vi "Excel_Page_Setup.vi"(0 "Excel._Worksheet":refnum<k7>, 5 "Excel._Application":refnum<k7>, 7 "margins (1.00)":T1 {"bottom" format="%0.2f"; "right" format="%0.2f"; "left" format="%0.2f"; "top" format="%0.2f"}, 9 "measurement system (Default)":u16, 11 "error in (no error)":errorcluster) -> (15 "error out":errorcluster)   [LabVIEW 2017, in "NI_ReportGenerationToolkit.lvlib"]
uses:
  <vilib>/addons/_office/NI_ReportGenerationToolkit.lvlib
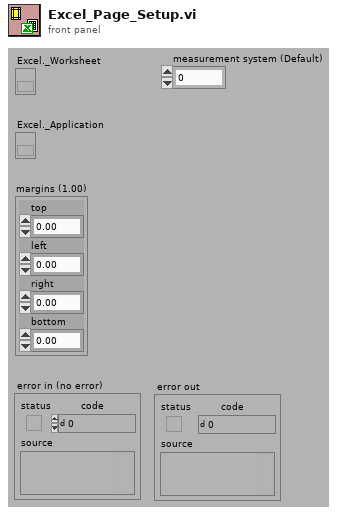
[diagram p1: front panel]
types:
  T1 = cluster{"top":dbl, "left":dbl, "right":dbl, "bottom":dbl}
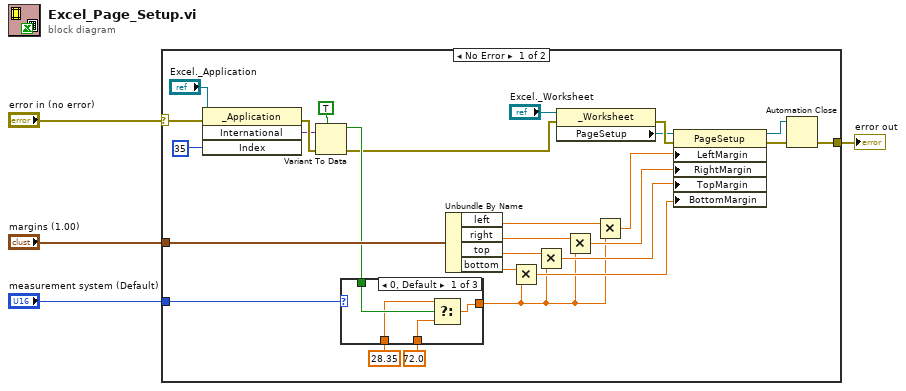
[diagram p0: block diagram]
diagram:
  n1 = case shown="No Error" "error in (no error)" {
    selector: "error in (no error)" -> [w5 w38]
    tunnel: "margins (1.00)" -> [w31 _]
    tunnel: "measurement system (Default)" -> [w11 _]
    tunnel: [w10 w38] -> w2
    frame No Error {
      n2 = invoke class="_Application" method="International"(reference="Excel._Application", error in=w5, "Index"=35) -> (error out=w21:errorcluster, "International"=w20:variant)  [unwired: 1 in, 2 out]
      n3 = Variant To Data(error in=w21, type=TRUE, Variant=w20) -> (data=w24:bool, error out=w22:errorcluster)
      n4 = case shown="0, Default" w11 {
        tunnel: [w35 w36 w37] -> w12
        tunnel: 72.0 -> [w32 w36 _]
        tunnel: w24 -> [w34 _ _]
        tunnel: 28.35 -> [w33 _ w37]
        frame 0, Default {
          n5 = Select(t=w33, s=w34, f=w32) -> (s? t:f=w35:dbl)
        }
        frame 1 {
        }
        frame 2 {
        }
      }
      n6 = Unbundle By Name(w31) -> ("left"=w30:dbl, "right"=w29:dbl, "top"=w28:dbl, "bottom"=w27:dbl)
      n7 = Multiply(x=w27, y=w12) -> (x*y=w16:dbl)
      n8 = Multiply(x=w28, y=w12) -> (x*y=w15:dbl)
      n9 = property class="_Worksheet"(reference="Excel._Worksheet", error in=w22) -> (error out=w9:errorcluster, "PageSetup"=w6:refnum<k7>)  [unwired: 1 out]
      n10 = Multiply(x=w29, y=w12) -> (x*y=w14:dbl)
      n11 = Multiply(x=w30, y=w12) -> (x*y=w13:dbl)
      n12 = property class="PageSetup"(reference=w6, error in=w9, "LeftMargin"=w13, "RightMargin"=w14, "TopMargin"=w15, "BottomMargin"=w16) -> (reference out=w7:refnum<k7>, error out=w8:errorcluster)
      n13 = Automation Close(3:w8, 5:w7) -> (0:w10:errorcluster)
    }
    frame Error {
    }
  }
  "error out" <- w2
